vi "Example 9 - Multi Tags.vi"() -> ()   [LabVIEW 2021]
uses:
  Omni-Bus/Omni_Bus.lvclass
  Omni-Bus/Support/Broad Types.ctl
  Local Bus/Local Bus.lvclass
  C:/Users/Tim/Documents/GitHub/Omni-Bus/Source/Omni-Bus/Bus Access/Bus_Access.lvclass
  Aggregator Bus/Aggregator Bus.lvclass
  <vilib>/Utility/Data Type/Type Definitions/Data Type.ctl
  <vilib>/TSA/Abstract Data Classes/Abs_Types/Type/Abs_Type.lvclass/Abs_Type.ctl
  Omni-Bus/Omni_Bus.lvclass/Omni_Bus.ctl
  Omni-Bus/Support/Write/Write Multi DBL.vi
  Omni-Bus/Support/Read/Read Multi DBL.vi
  Omni-Bus/Support/Get/Get Multi DBL.vi
  Omni-Bus/Support/FindMultiVar.vi
  Omni-Bus/Support/FindVar.vi
  <vilib>/Utility/error.llb/Clear Errors.vi
  Omni-Bus/Properties/Read Var Map.vi
  <vilib>/TSA/Abstract Data Classes/Abs_Types/Type/Properties/Read Tag.vi
  <vilib>/TSA/Abstract Data Classes/Constants/Support/DBL/Const_DBL.lvclass
  C:/Program Files (x86)/National Instruments/LabVIEW 2021/vi.lib/TSA/Abstract Data Classes/Abs_Types/Type/Abs_Type.lvclass
  <vilib>/TSA/Abstract Data Classes/Abs_Types/Double Float/Abs_Double Float.lvclass
  <vilib>/TSA/Abstract Data Classes/Abs_Types/Value/Abs_Value.lvclass
  <vilib>/TSA/Abstract Data Classes/Constants/Support/DBL/DBL.vi
  Omni-Bus/Support/Check For Read Only Error.vi
  Omni-Bus/Support/Incorrect Tag String Error.vi
  <vilib>/TSA/Abstract Data Classes/Abs_Types/Type/Abs_Type.lvclass
  <vilib>/Utility/Data Type/NI_Data Type.lvlib
panel:
  out "Read DBL error":errorcluster
  out "Write DBL error":errorcluster
  in  "Double":dbl[](array[numeric])
  in  "Write DBL Tag":string[](array[combo])
  in  "stop":bool
  out "Double":dbl[](array[numeric]) format="%.2f"
  in  "Read DBL Tag":string[](array[combo])
  out "error out":errorcluster
  out "All Tags":string[](array[string])
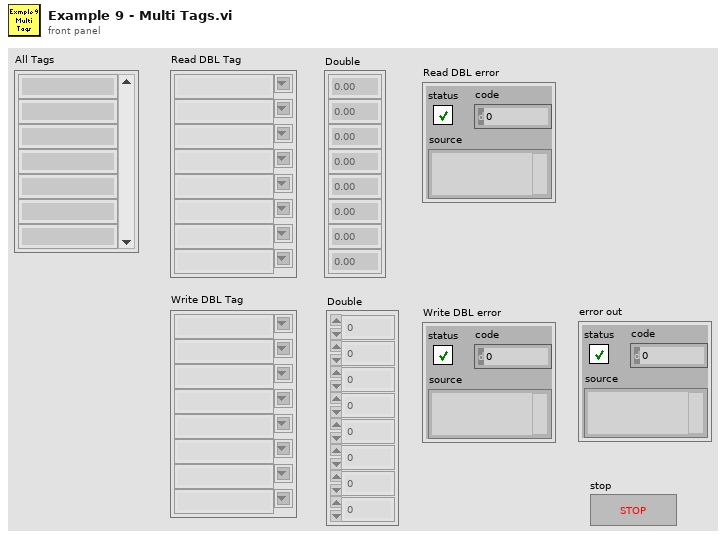
[diagram p1: front panel]
types:
  T1 = typedef "NI_Data Type.lvlib/Data Type.ctl" = enum8{"Invalid Type", "Void", "I8", "I16", "I32", "I64", "U8", "U16", "U32", "U64", "Single Float", "Double Float", "Extended Float", "Single Complex", "Double Complex", "Extended Complex", "Enum U8", "Enum U16", "Enum U32", "Enum U64", "Single Float With Unit", "Double Float With Unit", "Extended Float With Unit", "Single Complex with Unit", "Double Complex with Unit", "Extended Complex with Unit", "Boolean", "String", "Path", "Picture", "Tag", "Array", "Cluster", "Variant", "LV Variant", "Waveform", "Timestamp", "Digital Waveform", "Digital Data", "ExpressData", "Refnum", "External Data", "VI", "Poly VI", "LabVIEW Class Instance", "Fixed Point", "Set Collection", "Map Collection"}
  T2 = typedef "Omni_Bus.lvclass/Broad Types.ctl" = enum16{"All Tags", "NI Specific Type", "Boolean", "String", "Numeric", "Float", "Integer", "Collection", "All Value Types", "Non Value Types"}
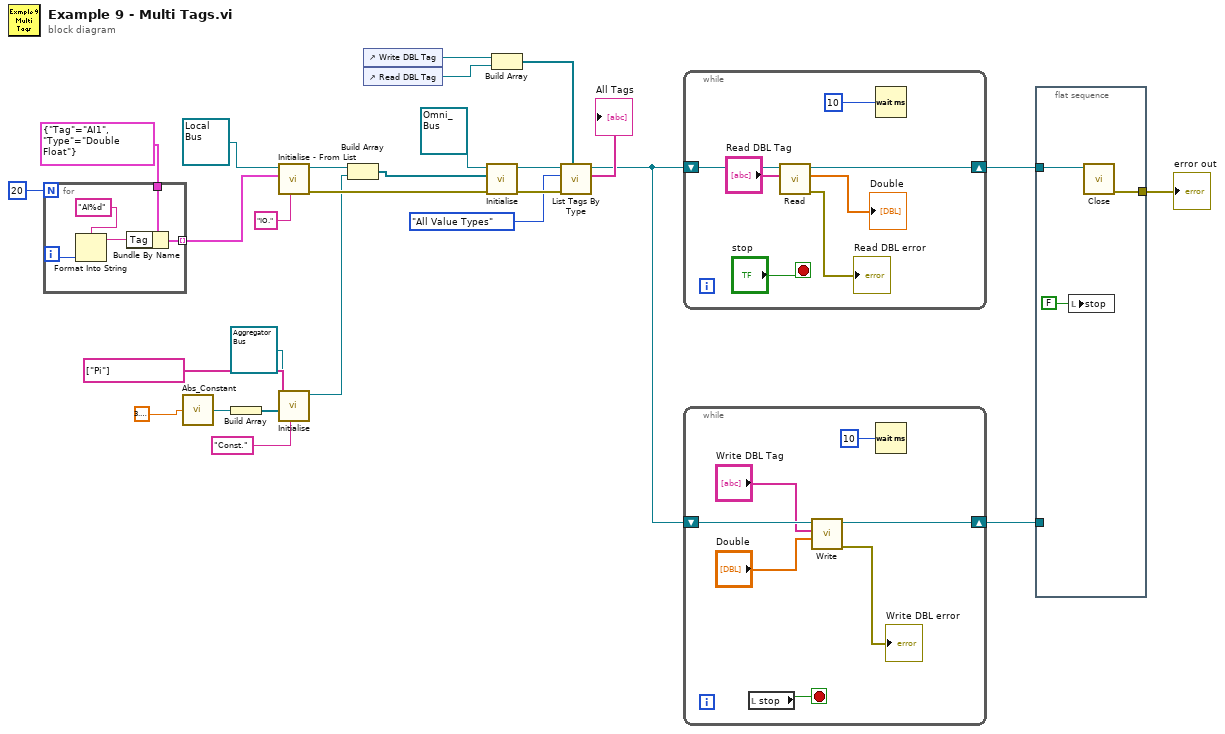
[diagram p0: block diagram]
diagram:
  n1 = for {
    N: 20 -> [_]
    tunnel: cluster{"Tag":string, "Type":T1} {"Tag"="AI1", "Type"=enum."Double Float"} ("Cluster") -> [w30]
    tunnel: [w28] -> w2 mode=indexing
    i -> [w31]
    n2 = Format Into String(format string="AI%d" ("Tag"), w31) -> (resulting string=w29:string)  [unwired: 2 in, 1 out]
    n3 = Bundle By Name(cluster=w30, "Tag"=w29) -> (w28:cluster{"Tag":string, "Type":T1})
  }
  n4 = call-poly <vilib>:"Abs_Constant.vi"("Value"=3.141592653589793) -> ("Constant"=w13:refnum<class "Const_DBL.lvclass">)  [unwired: 4 in]
  n5 = Build Array(w13) -> (w14:refnum<class "Const_DBL.lvclass">[])
  n6 = call "Initialise - From List.vi"("Tag Root"="IO.", "Tag List"=w2, "Local Bus in"=refnum<class "Local Bus.lvclass"> refnum ("Local Bus.lvclass")) -> ("error out"=w16:errorcluster, "Local Bus out"=w18:refnum<class "Local Bus.lvclass">)  [unwired: 7 in]
  n7 = call "Initialise.vi"("Tag Root"="Const.", "Values"=w14, "Tags"=string[] ["Pi"], "Aggregator Bus in"=refnum<class "Aggregator Bus.lvclass"> refnum) -> ("Aggregator Bus out"=w15:refnum<class "Aggregator Bus.lvclass">)  [unwired: 6 in, 1 out]
  n8 = Build Array(w18, w15) -> (w4:refnum<class "Bus_Access.lvclass">[])
  n9 = control-ref of="Write DBL Tag"() -> (w9:refnum<vi>)
  n10 = control-ref of="Read DBL Tag"() -> (w8:refnum<vi>)
  n11 = call-dynamic "Initialise.vi"("error in (no error)"=w16, "Bus Access"=w4, "Var Bus in"=refnum<class "Omni_Bus.lvclass"> refnum) -> ("error out"=w25:errorcluster, "Var Bus out"=w26:refnum<class "Omni_Bus.lvclass">)  [unwired: 7 in]
  n12 = Build Array(w9, w8) -> (w7:refnum<vi>[])
  n13 = call "List Tags By Type.vi"("Combo Boxes"=w7, "error in (no error)"=w25, "Broad Types"=Broad_Types."All Value Types", "Var Bus in"=w26) -> ("Tags"=→"All Tags":string[], "Var Bus out"=w20:refnum<class "Omni_Bus.lvclass">)  [unwired: 4 in, 2 out]
  n14 = while {
    shift-right: [w33] -> w21
    shift-left: w20 -> [w39]
    stop <- "stop" stop-if-true
    n15 = call-poly "Read.vi"("Tag"="Read DBL Tag", "Var Bus in"=w39) -> ("error out"=→"Read DBL error":errorcluster, "DBL's"=→"Double":dbl[], "Var Bus out"=w33:refnum<class "Omni_Bus.lvclass">)  [unwired: 7 in]
    n16 = Wait (ms)(milliseconds to wait=u32 10) -> ()  [unwired: 1 out]
  }
  n17 = while {
    shift-right: [w40] -> w19
    shift-left: w20 -> [w46]
    stop <- w43 stop-if-true
    n18 = local read "stop"() -> (w43:bool)
    n19 = call-poly "Write.vi"("Array"="Double", "Tag"="Write DBL Tag", "Omni_Bus in"=w46) -> ("error out"=→"Write DBL error":errorcluster, "Omni_Bus out"=w40:refnum<class "Omni_Bus.lvclass">)  [unwired: 7 in]
    n20 = Wait (ms)(milliseconds to wait=u32 10) -> ()  [unwired: 1 out]
  }
  n21 = flat-sequence {
    tunnel: [w49] -> w22
    tunnel: w21 -> [w48]
    tunnel: w19 -> [_]
    frame #0 {
      n22 = local write "stop"(FALSE ("stop")) -> ()
      n23 = call-dynamic "Close.vi"("Data in"=w48) -> ("error out"=w49:errorcluster)  [unwired: 9 in, 1 out]
    }
  }
  "error out" <- w22
